vi "Generate Simulated Data.vi"(7 "Type de mode":bool, 8 "error in (no error)":T2 caption="entrée d'erreur (pas d'erreur)", 9 "Péri":tag="Dev1", 10 "Longueur d'onde":dbl, 11 "Type de signal":T1) -> (0 "error out":T2 caption="sortie d'erreur", 2 "Données du graphe":waveform(dbl)[](array[waveform]))   [LabVIEW 2018, in "Acquisition.lvlib"]
doc: "Génère des exemples de waveforms en fonction du type de signal dans l'entrée Configuration du matériel."
uses:
  Acquisition.lvlib
  Signal Type.ctl
  <vilib>/Analysis/NI_AALBase.lvlib
panel:
  out "Graphe déroulant":dynamicdata(graph)
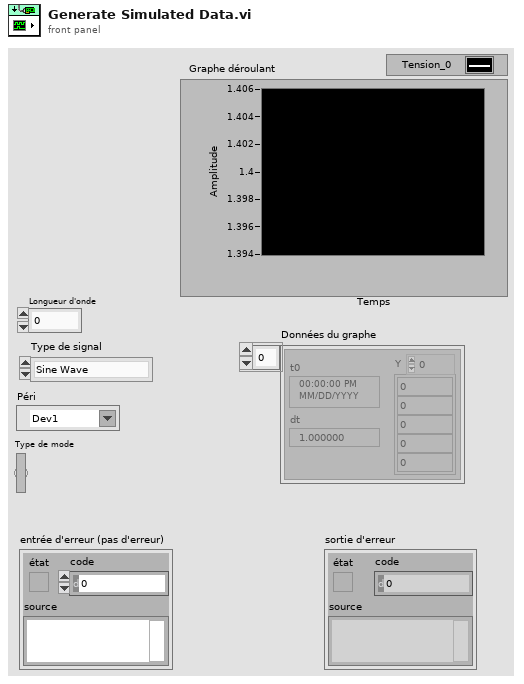
[diagram p1: front panel]
types:
  T1 = typedef "Acquisition.lvlib/Signal Type.ctl" = enum16{"Sine Wave", "Square with Noise", "Signal triangulaire", "Simulation DAQ"}
  T2 = cluster{"état":bool, "code":i32, "source":string}
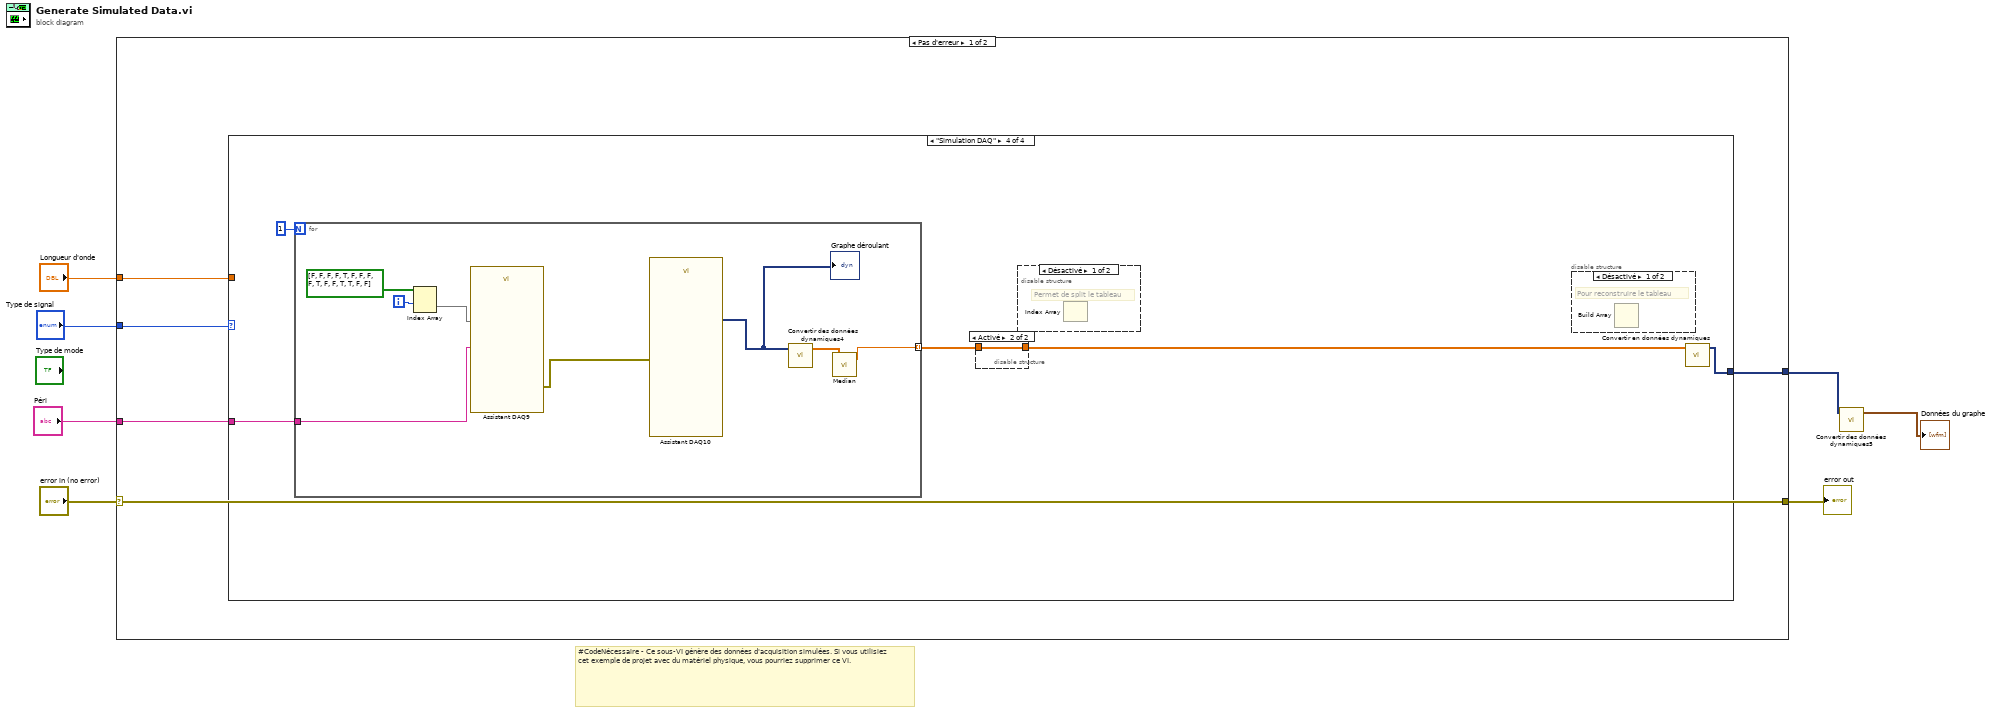
[diagram p0: block diagram]
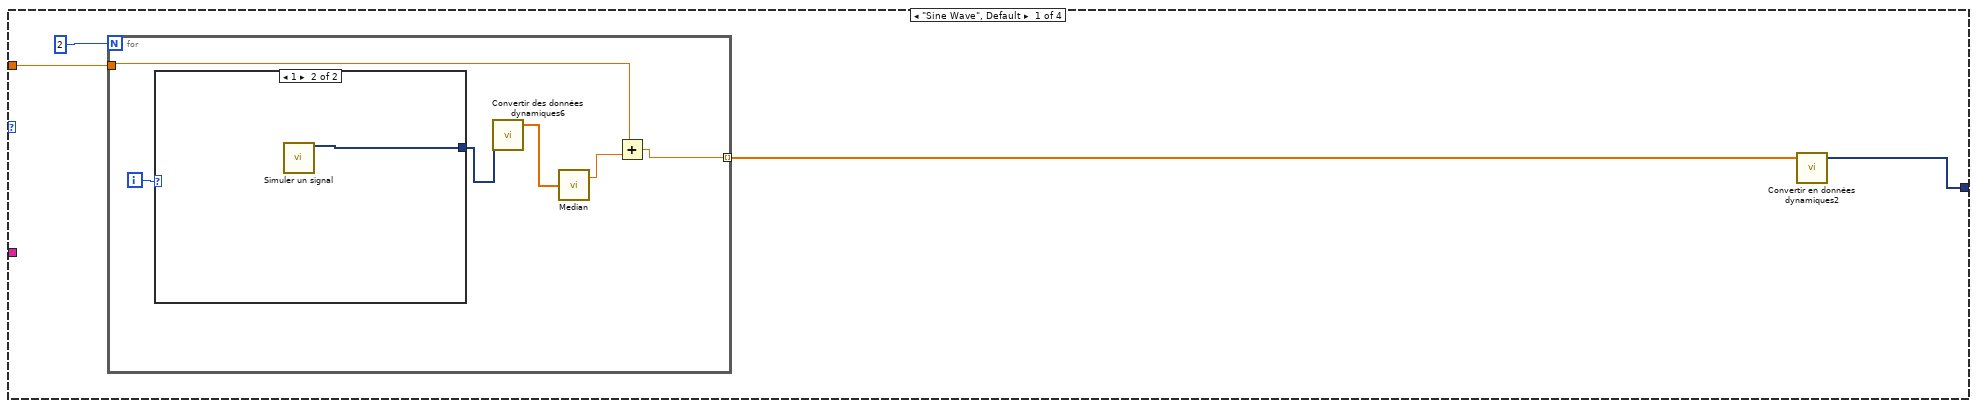
[diagram p2: hidden frame]
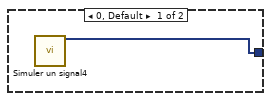
[diagram p3: hidden frame]
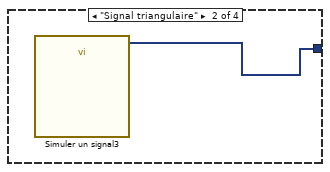
[diagram p4: hidden frame]
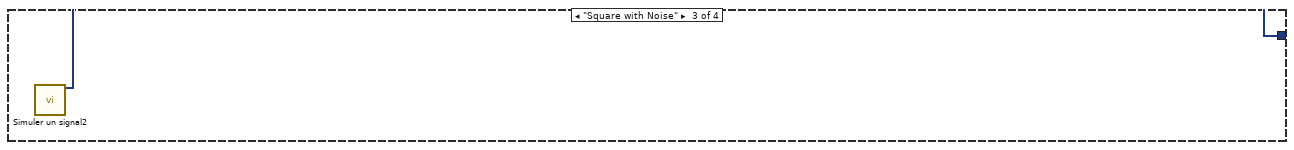
[diagram p5: hidden frame]
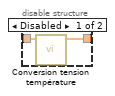
[diagram p6: hidden frame]
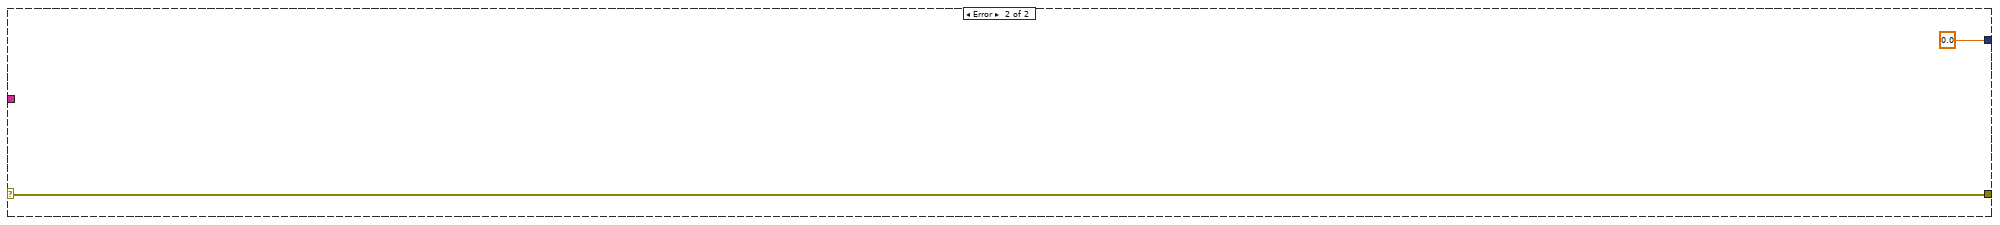
[diagram p9: hidden frame]
diagram:
  # "#CodeNécessaire - Ce sous-VI génère des données d'acquisition simulées. Si vous utilisiez cet exemple de projet avec du matériel physique, vous pourriez supprimer ce VI."
  n1 = case shown="Pas d'erreur" "error in (no error)" {
    selector: "error in (no error)" -> [w12 w44]
    tunnel: [w12 w44] -> w6
    tunnel: "Type de signal" -> [w11 _]
    tunnel: [w10 0.0] -> w3
    tunnel: "Longueur d'onde" -> [w9 _]
    tunnel: "Péri" -> [w8 _]
    frame No Error {
      n2 = case shown="\"Simulation DAQ\"" w11 {
        tunnel: [w15 w25 w26 w30] -> w10
        tunnel: w9 -> [w14 _ _ _]
        tunnel: w8 -> [_ _ _ w29]
        frame "Sine Wave", Default {
          n3 = for {
            N: 2 -> [_]
            tunnel: [w18] -> w13 mode=indexing
            tunnel: w14 -> [w17]
            i -> [w22]
            n4 = case shown="1" w22 {
              tunnel: [w23 w24] -> w21
              frame 0, Default {
                n5 = call "Simuler un signal4"() -> ("CC"=w23:dynamicdata)  [unwired: 14 in, 1 out]
              }
              frame 1 {
                n6 = call "Simuler un signal"() -> ("Sinus avec Bruit uniforme"=w24:dynamicdata)  [unwired: 14 in, 1 out]
              }
            }
            n7 = call "Convertir des données dynamiques6"("Dynamic Data Type"=w21) -> ("Array"=w20:dbl[])  [unwired: 3 in]
            n8 = call <vilib>:"Median.vi"("X"=w20) -> ("median"=w19:dbl)  [unwired: 1 out]
            n9 = Add(x=w17, y=w19) -> (x+y=w18:dbl)
          }
          n10 = call "Convertir en données dynamiques2"("Array"=w13) -> ("Dynamic Data Type"=w15:dynamicdata)  [unwired: 3 in]
        }
        frame "Signal triangulaire" {
          n11 = call "Simuler un signal3"() -> ("Triangle"=w25:dynamicdata)  [unwired: 14 in, 1 out]
        }
        frame "Square with Noise" {
          n12 = call "Simuler un signal2"() -> ("Square with Gaussian Noise"=w26:dynamicdata)  [unwired: 14 in, 1 out]
        }
        frame "Simulation DAQ" {
          n13 = for {
            N: 1 -> [_]
            tunnel: [w42] -> w28 mode=indexing
            tunnel: w29 -> [w35]
            i -> [w37]
            n14 = Index Array(array=bool[][] [[FALSE, FALSE, FALSE, FALSE], [TRUE, FALSE, FALSE, FALSE], [FALSE, TRUE, FALSE, FALSE], [TRUE, TRUE, FALSE, FALSE]], index (row)=w37) -> (element=w36:bool[])  [unwired: 1 in]
            n15 = call "Assistant DAQ9"("data"=w36, "nom du périphérique"=w35) -> ("error out"=w40:errorcluster)  [unwired: 16 in, 1 out]
            n16 = call "Assistant DAQ10"("error in"=w40) -> ("data"=w39:dynamicdata)  [unwired: 16 in, 2 out]
            "Graphe déroulant" <- w39
            n17 = call "Convertir des données dynamiques4"("Dynamic Data Type"=w39) -> ("Array"=w41:dbl[])  [unwired: 3 in]
            n18 = call <vilib>:"Median.vi"("X"=w41) -> ("median"=w42:dbl)  [unwired: 1 out]
          }
          n19 = disable-structure shown="Activé" {
            disable-tunnel: w28 -> [w33 w34]
            disable-tunnel: [w32 w34] -> w27
            frame Disabled {
              n20 = call "Conversion tension température.vi"("Data In"=w33) -> ("Data Out"=w32:dbl[])  [unwired: 10 in]
            }
            frame Enabled {
            }
          }
          n21 = disable-structure shown="Désactivé" {
            frame Disabled {
              # "Permet de split le tableau"
              n22 = Index Array() -> ()  [unwired: 2 in, 1 out]
            }
            frame Enabled {
            }
          }
          n23 = disable-structure shown="Désactivé" {
            frame Disabled {
              # "Pour reconstruire le tableau"
              n24 = Build Array() -> ()  [unwired: 4 in, 1 out]
            }
            frame Enabled {
            }
          }
          n25 = call "Convertir en données dynamiques"("Array"=w27) -> ("Dynamic Data Type"=w30:dynamicdata)  [unwired: 3 in]
        }
      }
    }
    frame Error {
    }
  }
  "error out" <- w6
  n26 = call "Convertir des données dynamiques5"("Dynamic Data Type"=w3) -> ("Array of Waveform"=→"Données du graphe":waveform(dbl)[])  [unwired: 3 in]
